vi "Read Value.vi"(8 "error in (no error)":errorcluster, 11 "AISAS motor in":refnum<class "AISAS motor.lvclass">) -> (0 "error out":errorcluster, 2 "Value":variant, 3 "AISAS motor out":refnum<class "AISAS motor.lvclass">)   [LabVIEW 2014, in "AISAS motor.lvclass"]
uses:
  AISAS motor.lvclass
  AISAS motor.lvclass/AISAS motor.ctl
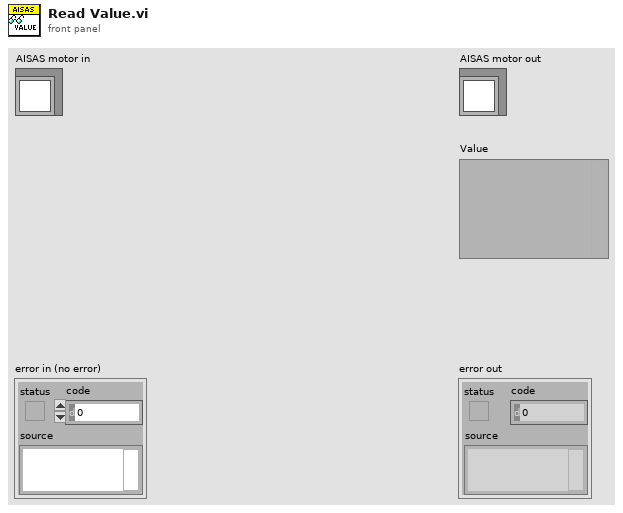
[diagram p1: front panel]
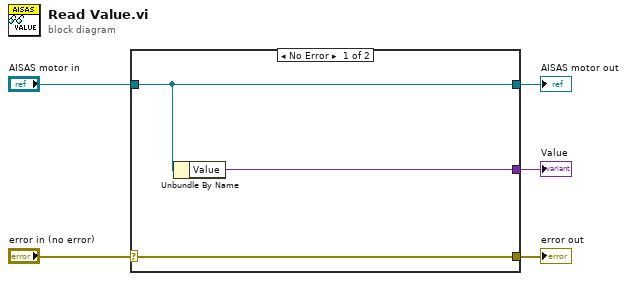
[diagram p0: block diagram]
diagram:
  n1 = case shown="No Error" "error in (no error)" {
    selector: "error in (no error)" -> [w8 w9]
    tunnel: [w8 w9] -> w4
    tunnel: [w7 w10] -> w2
    tunnel: "AISAS motor in" -> [w7 w10]
    tunnel: [w6 _] -> w1
    frame No Error {
      n2 = Unbundle By Name(w7) -> ("Value"=w6:variant)
    }
    frame Error {
    }
  }
  "error out" <- w4
  "AISAS motor out" <- w2
  "Value" <- w1
